vi "Principal.vi"() -> ()   [LabVIEW 2014]
panel:
  out "index of element":i32
  in  "stopButton":bool
  in  "startButton":bool
  in  "exitButton":bool
  out "Cluster":T1={"confGeralButton"=TRUE, "calibraButton"=FALSE, "ensaioButton"=FALSE}
  out "ledVibracao":bool caption="Vibração"
  out "ledCarga":bool caption="Célula"
  out "ledRotacao":bool caption="Rotação"
  out "ledTermoparRef":bool caption="Termopar Ref"
  out "ledTermoparB":bool caption="Termopar B"
  out "ledTermoparA":bool caption="Termopar A"
  in  "pathToFile":path
  in  "Boolean 2":bool
  in  "Boolean":bool
  out "Freio":bool
  out "Motor":bool
  # "-"
  # "001"
  # "999"
  # "Bancada de Frenagem - Ensaio"
  # "Sensores"
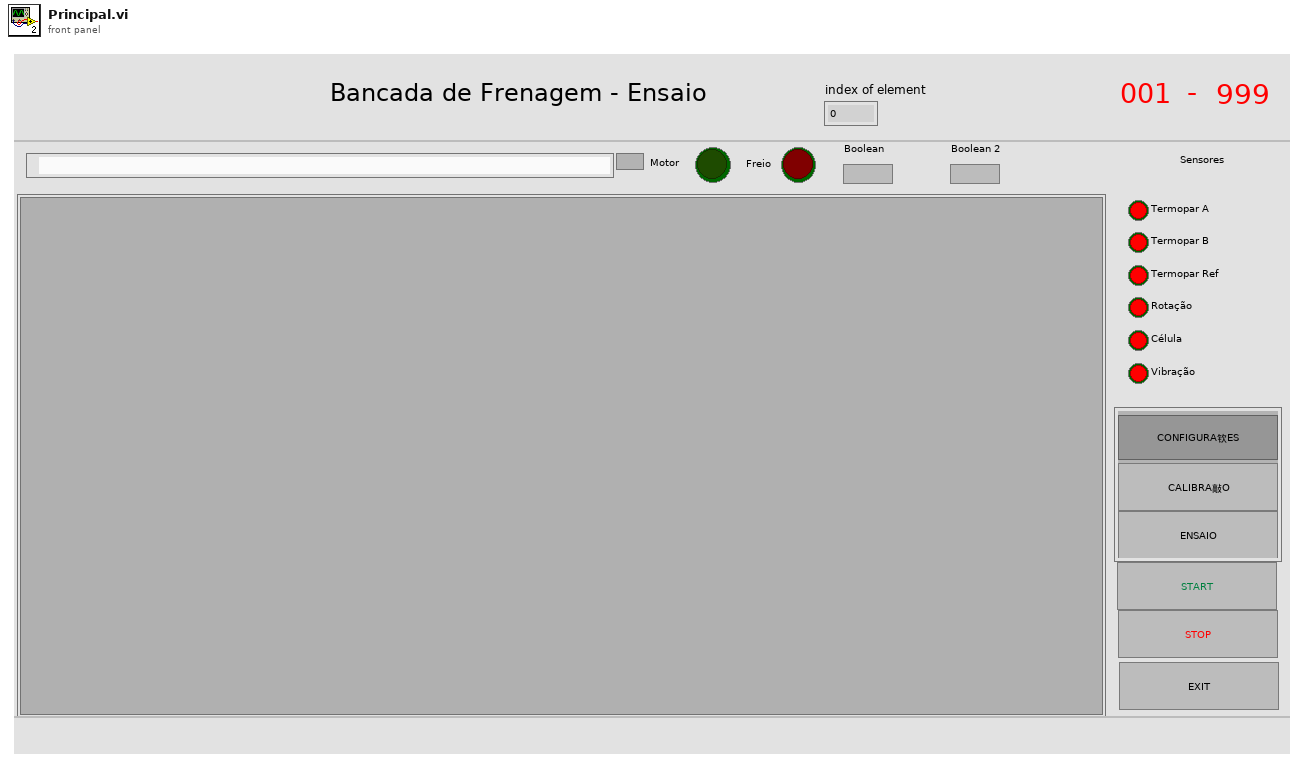
[diagram p1: front panel]
types:
  T1 = cluster{"confGeralButton":bool, "calibraButton":bool, "ensaioButton":bool}
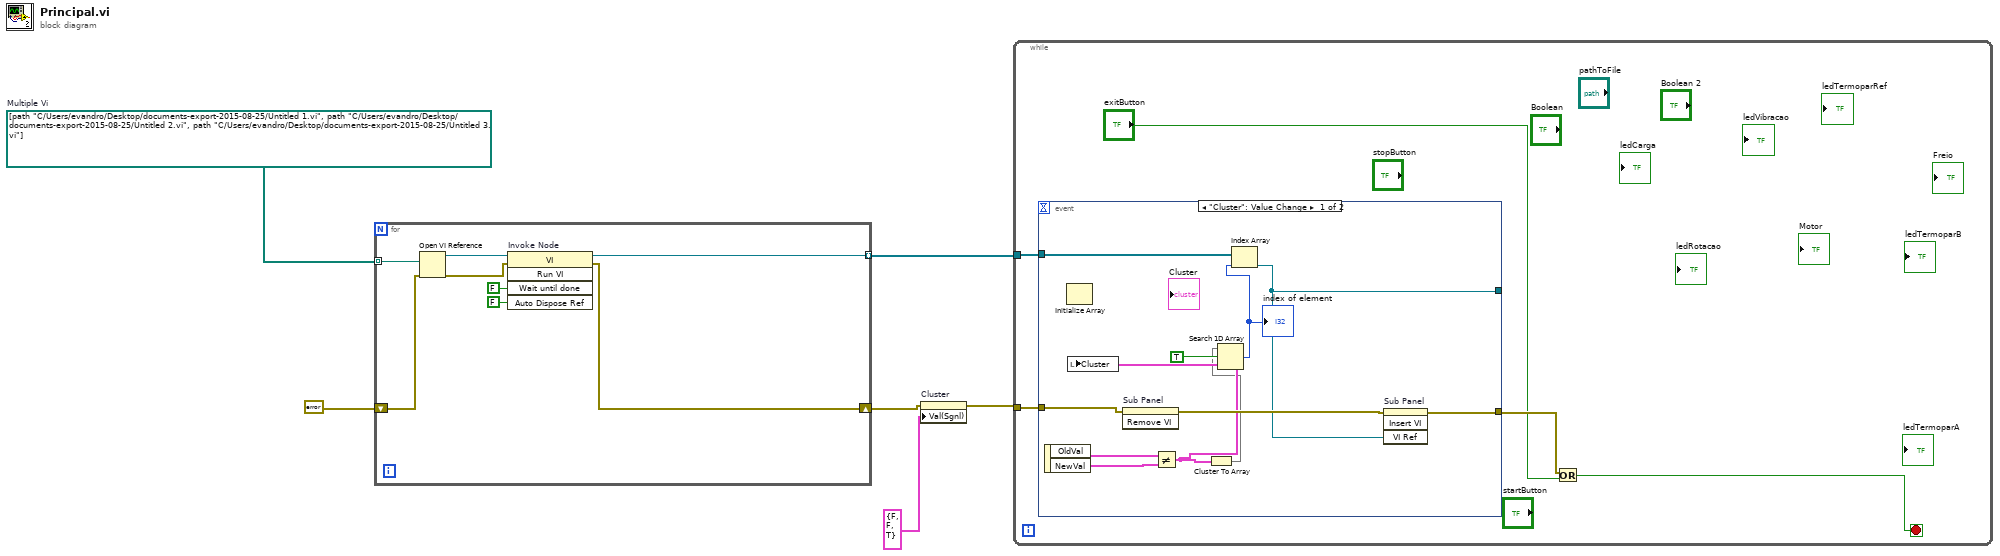
[diagram p0: block diagram]
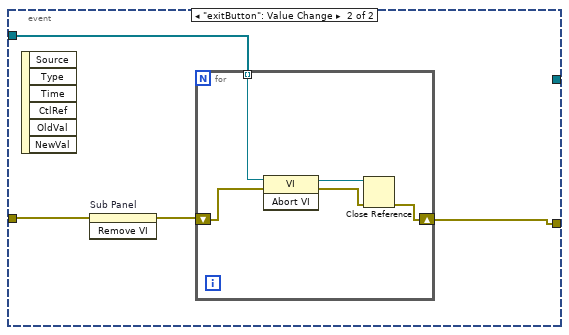
[diagram p2: hidden frame]
diagram:
  w6 = path[] [path "C:/Users/evandro/Desktop/documents-export-2015-08-25/Untitled 1.vi", path "C:/Users/evandro/Desktop/documents-export-2015-08-25/Untitled 2.vi", path "C:/Users/evandro/Desktop/documents-export-2015-08-25/Untitled 3.vi"]  # Multiple Vi
  n1 = for {
    tunnel: w6 -> [w14] mode=indexing
    shift-right: [w12] -> w3
    shift-left: errorcluster {FALSE, 0, ""} -> [w7]
    tunnel: [w11] -> w5 mode=indexing
    n2 = Open VI Reference(vi path=w14, error in (no error)=w7) -> (vi reference=w13:refnum<vi>, error out=w8:errorcluster)  [unwired: 4 in]
    n3 = invoke on="Invoke Node" class="VI" method="Run VI"(reference=w13, error in=w8, "Wait until done"=FALSE ("Wait Until Done"), "Auto Dispose Ref"=FALSE ("Auto Dispose Reference")) -> (reference out=w11:refnum<vi>, error out=w12:errorcluster)  [unwired: 1 in, 3 out]
  }
  n4 = property on="Cluster" class="Clust (strict)"(error in=w3, "Val(Sgnl)"=T1 {"confGeralButton"=FALSE, "calibraButton"=FALSE, "ensaioButton"=TRUE} ("Value (Signaling)")) -> (error out=w4:errorcluster)  [unwired: 1 in, 1 out]
  n5 = while {
    tunnel: w5 -> [w18]
    tunnel: w4 -> [w19]
    stop <- w15 stop-if-true
    n6 = event shown="[0] \"Cluster\": Value Change" {
      selector: _ -> [_ _]
      dyn-events: _ -> [_ _]
      timeout: _ -> [_ _]
      tunnel: w19 -> [w30 w32]
      tunnel: w18 -> [w28 w34]
      tunnel: [w27 w31] -> w17
      tunnel: [w26 _] -> _
      event "Cluster": Value Change {
        n7 = event-data() -> ("OldVal"=w25:T1, "NewVal"=w24:T1)  [unwired: 1 in]
        n8 = Initialize Array() -> ()  [unwired: 2 in, 1 out]
        n9 = invoke on="Sub Panel" class="SubPnl" method="Remove VI"(error in=w30) -> (error out=w29:errorcluster)  [unwired: 2 in, 2 out]
        n10 = Not Equal?(x=w25, y=w24) -> (x != y?=w21:T1)
        n11 = local write "Cluster"(w21) -> ()
        n12 = Cluster To Array(cluster=w21) -> (array=w20:bool[])
        n13 = Search 1D Array(1D array=w20, element=TRUE) -> (index of element=w23:i32)  [unwired: 1 in]
        "index of element" <- w23
        n14 = Index Array(array=w28, index=w23) -> (element=w26:refnum<vi>)
        n15 = invoke on="Sub Panel" class="SubPnl" method="Insert VI"(error in=w29, "VI Ref"=w26) -> (error out=w27:errorcluster)  [unwired: 2 in, 3 out]
      }
      event "exitButton": Value Change {
        n16 = event-data() -> ()  [unwired: 1 in, 6 out]
        n17 = invoke on="Sub Panel" class="SubPnl" method="Remove VI"(error in=w32) -> (error out=w33:errorcluster)  [unwired: 2 in, 2 out]
        n18 = for {
          tunnel: w34 -> [w39] mode=indexing
          shift-right: [w35] -> w31
          shift-left: w33 -> [w36]
          n19 = invoke class="VI" method="Abort VI"(reference=w39, error in=w36) -> (reference out=w38:refnum<vi>, error out=w37:errorcluster)  [unwired: 1 in, 1 out]
          n20 = Close Reference(reference=w38, error in (no error)=w37) -> (error out=w35:errorcluster)
        }
      }
    }
    n21 = Or(x=w17, y="exitButton") -> (x .or. y?=w15:bool)
  }
